vi "ScaleLink.vi"(7 "首次调用":bool, 8 "曲线输入":dbl[][](array[numeric]), 11 "通量输入":dbl[](array[numeric])) -> (0 "开启衔接指示":bool, 3 "通量输出":dbl[](array[numeric]))   [LabVIEW 2020]
uses:
  <vilib>/Analysis/polynomials.llb/Scalar Polynomial Evaluation (DBL).vi
  <vilib>/Analysis/NI_AALPro.lvlib
panel:
  out "量程衔接曲线":dbl[][](graph)
  in  "待接量程":u16(ring) items=["电压7", "电压8", "电流1", "电流2"]
  in  "子量程":u16(ring) items=["电压7", "电压8", "电流1", "电流2"]
  out "待接量程当前值":dbl
  out "子量程当前值":dbl
  in  "开关":bool caption="开启衔接："
  out "衔接系数":dbl[](array[numeric]) min=0.0 max=127.0 format="%#.2f"
  out "最新衔接值":dbl caption="最新衔接值："
  in  "通量名称":string[](array[string])
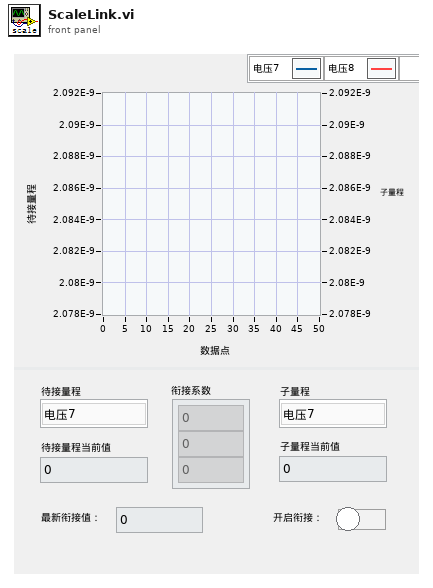
[diagram p1: front panel]
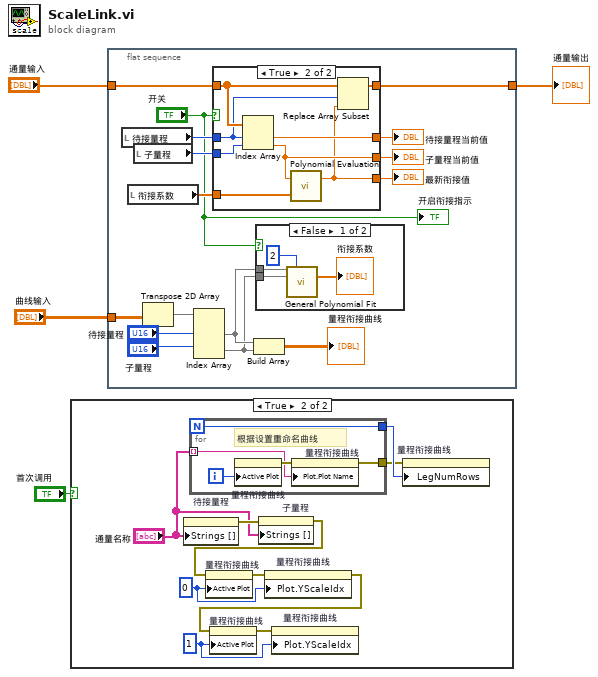
[diagram p0: block diagram]
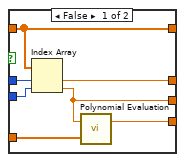
[diagram p4: hidden frame]
diagram:
  n1 = case shown="True" "首次调用" {
    frame False {
    }
    frame True {
      w12 = u32 1 ("活动曲线")
      w13 = u32 0 ("活动曲线")
      n2 = property on="待接量程" class="Ring (strict)"("Strings []"="通量名称") -> (error out=w9:errorcluster)  [unwired: 2 in, 1 out]
      n3 = for {
        N -> [w16]
        tunnel: "通量名称" -> [w17] mode=indexing
        tunnel: [w16] -> w8
        tunnel: [w15] -> w7
        i -> [w19]
        # "根据设置重命名曲线"
        n4 = property on="量程衔接曲线" class="WFGraph (strict)"("Active Plot"=w19) -> (error out=w18:errorcluster)  [unwired: 2 in, 1 out]
        n5 = property on="量程衔接曲线" class="WFGraph (strict)"(error in=w18, "Plot.Plot Name"=w17) -> (error out=w15:errorcluster)  [unwired: 1 in, 1 out]
      }
      n6 = property on="子量程" class="Ring (strict)"(error in=w9, "Strings []"="通量名称") -> (error out=w14:errorcluster)  [unwired: 1 in, 1 out]
      n7 = property on="量程衔接曲线" class="WFGraph (strict)"(error in=w14, "Active Plot"=w13) -> (error out=w6:errorcluster)  [unwired: 1 in, 1 out]
      n8 = property on="量程衔接曲线" class="WFGraph (strict)"(error in=w6, "Plot.YScaleIdx"=w13) -> (error out=w11:errorcluster)  [unwired: 1 in, 1 out]
      n9 = property on="量程衔接曲线" class="WFGraph (strict)"(error in=w11, "Active Plot"=w12) -> (error out=w10:errorcluster)  [unwired: 1 in, 1 out]
      n10 = property on="量程衔接曲线" class="WFGraph (strict)"(error in=w10, "Plot.YScaleIdx"=w12) -> ()  [unwired: 1 in, 2 out]
      n11 = property on="量程衔接曲线" class="WFGraph (strict)"(error in=w7, "LegNumRows"=w8) -> ()  [unwired: 1 in, 2 out]
    }
  }
  n12 = flat-sequence {
    tunnel: "通量输入" -> [w35]
    tunnel: [w34] -> w2
    tunnel: "曲线输入" -> [w21]
    frame #0 {
      n13 = local read "待接量程"() -> (w31:u16)
      n14 = local read "衔接系数"() -> (w27:dbl[])
      n15 = local read "子量程"() -> (w30:u16)
      n16 = Transpose 2D Array(2D array=w21) -> (transposed array=w20:dbl[][])
      n17 = Index Array(array=w20, index (row) #1="待接量程", index (row) #2="子量程") -> (element #1=w26:dbl[], element #2=w25:dbl[])  [unwired: 2 in]
      n18 = case shown="True" "开关" {
        tunnel: w35 -> [w44 w54]
        tunnel: [w44 w51] -> w34
        tunnel: w31 -> [w46 w53]
        tunnel: w30 -> [w45 w52]
        tunnel: [w43 w50] -> w29
        tunnel: [w41 w48] -> w28
        tunnel: w27 -> [w42 w49]
        tunnel: [w40 w47] -> w23
        frame False {
          n19 = Index Array(array=w44, index #1=w46, index #2=w45) -> (element #1=w43:dbl, element #2=w41:dbl)
          n20 = call-poly <vilib>:"Polynomial Evaluation.vi"("P(x)"=w42, "a"=w41) -> ("P(a)"=w40:dbl)  [unwired: 1 out]
        }
        frame True {
          n21 = Index Array(array=w54, index #1=w53, index #2=w52) -> (element #1=w50:dbl, element #2=w48:dbl)
          n22 = call-poly <vilib>:"Polynomial Evaluation.vi"("P(x)"=w49, "a"=w48) -> ("P(a)"=w47:dbl)  [unwired: 1 out]
          n23 = Replace Array Subset(array=w54, new element=w47, index=w53) -> (w51:dbl[])
        }
      }
      "待接量程当前值" <- w29
      "子量程当前值" <- w28
      "最新衔接值" <- w23
      n24 = Build Array(w26, w25) -> (→"量程衔接曲线":dbl[][])
      n25 = case shown="False" "开关" {
        tunnel: w26 -> [w39 _]
        tunnel: w25 -> [w38 _]
        frame False {
          n26 = call <vilib>:"General Polynomial Fit.vi"("Y"=w39, "polynomial order"=2, "X"=w38) -> ("Polynomial Coefficients"=→"衔接系数":dbl[])  [unwired: 9 in, 3 out]
        }
        frame True {
        }
      }
      "开启衔接指示" <- "开关"
    }
  }
  "通量输出" <- w2
